vi "Panel.vi"(11 "StokePlotShortcuts in":refnum<class "RocketPlotShortcuts.lvclass">) -> ()   [LabVIEW 2021, in "RocketPlot.lvlib" / "RocketPlotShortcuts.lvclass"]
uses:
  RocketPlotShortcuts.lvclass
  C:/Program Files/National Instruments/LabVIEW 2021/user.lib/bjustice/TipStripOOPanel/Classes/TipPanel/TipPanel.lvclass
  C:/Program Files/National Instruments/LabVIEW 2021/vi.lib/IlluminatedG/IG OOPanel/OOPanel/Panel/Panel.lvclass
  <userlib>/bjustice/TipStripOOPanel/Classes/TipPanel/TipPanel.lvclass/TipPanel.ctl
  <userlib>/bjustice/TipStripOOPanel/Classes/TipPanel/Read New Panel UE.vi
  <vilib>/Futures/Futures/Promise/Promise.lvclass
  RocketPlotShortcuts.lvclass/RocketPlotShortcuts.ctl
  <vilib>/IlluminatedG/IG OOPanel/OOPanel/Panel/Panel.lvclass
  <userlib>/bjustice/TipStripOOPanel/Classes/TipPanel/TipPanel.lvclass
  <vilib>/IlluminatedG/IG OOPanel/OOPanel/OOPanel.lvlib
panel:
  # "Autosize\nall axes"
  # "Zoom in\ntime axis"
  # "Page\nUp"
  # "Zoom in\ny axis"
  # "Home"
  # "Insert"
  # "Right Click"
  # "Delta values"
  # "Middle Click"
  # "Right Click +Ctrl"
  # "Slive average"
  # "Pan"
  # "Left Click"
  # "Right Click +Shift"
  # "Plot names"
  # "Zoom out\ntime axis"
  # "Page\nDown"
  # "Zoom out\ny axis"
  # "Delete"
  # "Zoom to\nselection"
  # "Tool Tips"
  # "Wheel scroll"
  # "Zoom in/out"
  # "Pan\nin increments"
  # "Zoom actions apply\nto all axes"
  # "Shift"
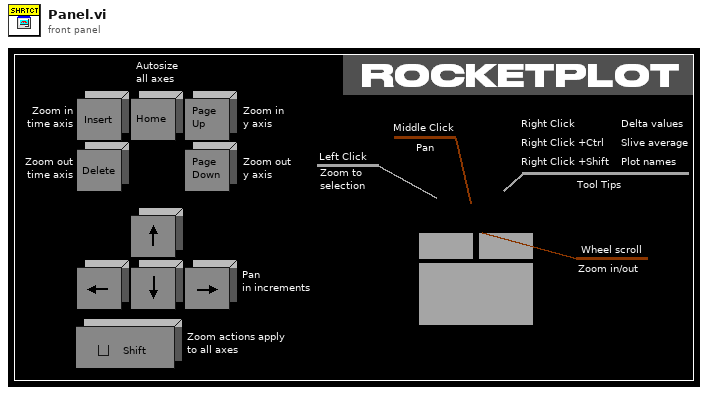
[diagram p1: front panel]
types:
  T1 = typedef "LVBoundsTypeDef.ctl" = cluster{"Width":u32, "Height":u32}
  T2 = typedef "OOPanel.lvlib/Panel.lvclass/Panel Events.ctl" = cluster{"Visbility":refnum<user-event>, "Close":refnum<user-event>}
  T3 = typedef "OOPanel.lvlib/Visibility State.ctl" = enum16{"Idle", "Closed", "Hidden", "Visible", "Subpanel", "Hidden Subpanel"}
  T4 = typedef "TipStrip2.lvlib/TipPanel.lvclass/ToPanelUE.ctl" = cluster{"TipPanel":refnum<class>, "Promise.Size":refnum<class "Promise.lvclass">}
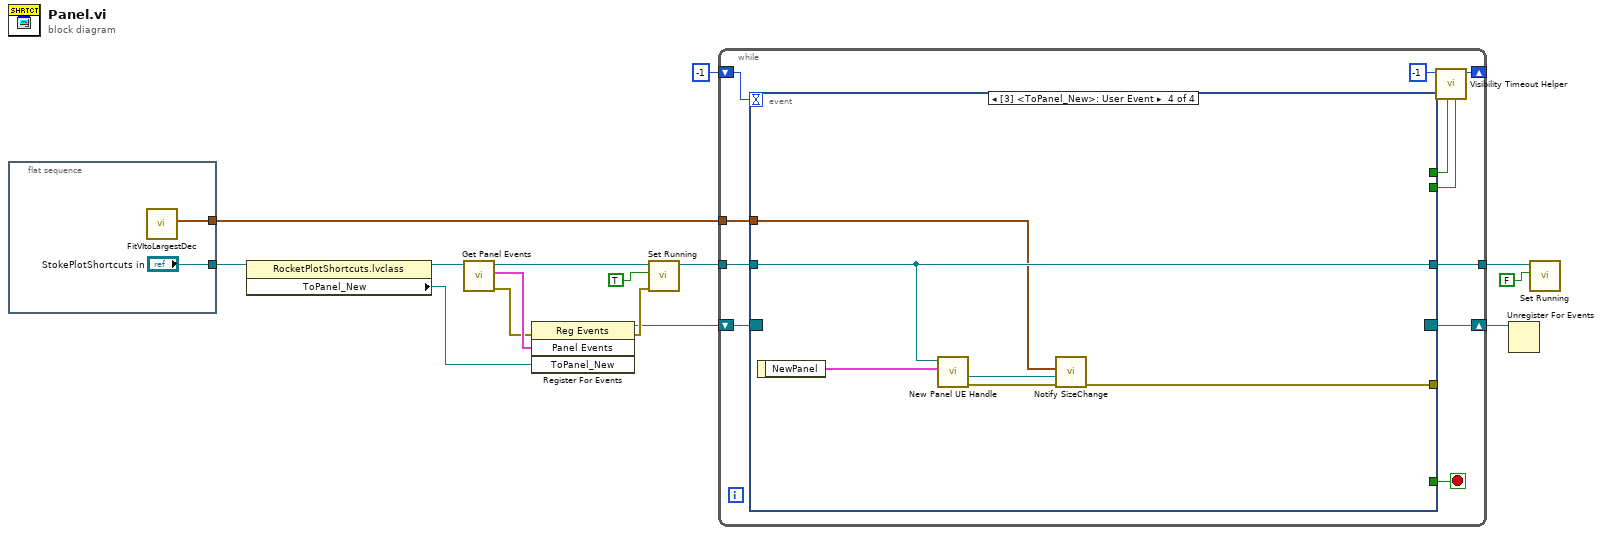
[diagram p0: block diagram]
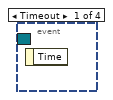
[diagram p2: hidden frame]
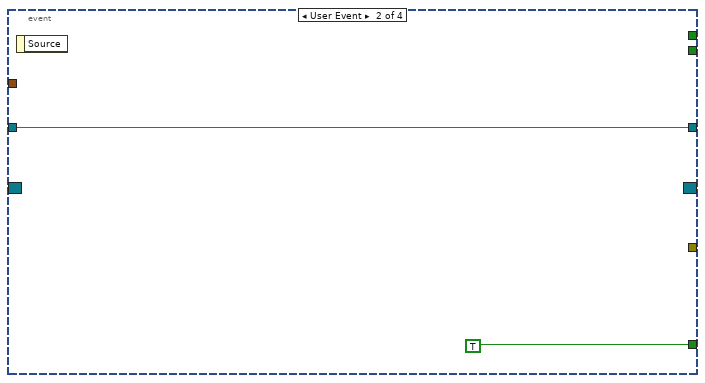
[diagram p3: hidden frame]
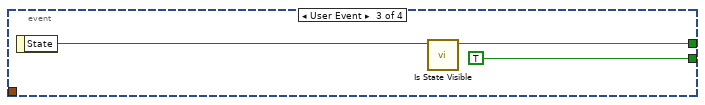
[diagram p4: hidden frame]
diagram:
  n1 = flat-sequence {
    tunnel: ["StokePlotShortcuts in"] -> w4
    tunnel: [w16] -> w1
    frame #0 {
      n2 = call "FitVItoLargestDec.vi"() -> ("content size"=w16:T1)  [unwired: 9 in, 2 out]
    }
  }
  n3 = property class="RocketPlotShortcuts.lvclass"(reference=w4) -> (reference out=w2:refnum<class "RocketPlotShortcuts.lvclass">, "ToPanel_New"=w3:refnum<user-event>)  [unwired: 1 in, 1 out]
  n4 = call <vilib>:"Get Panel Events.vi"("Panel in"=w2) -> ("error out"=w5:errorcluster, "Panel Events"=w15:T2, "Panel out"=w14:refnum<class "RocketPlotShortcuts.lvclass">)  [unwired: 8 in]
  n5 = register-events(error in=w5, w15, w3) -> (reference out=w11:refnum<event-registration>, error out=w12:errorcluster)  [unwired: 1 in]
  n6 = call <vilib>:"Set Running.vi"("error in (no error)"=w12, "Running"=TRUE, "Panel in"=w14) -> ("Panel out"=w10:refnum<class "RocketPlotShortcuts.lvclass">)  [unwired: 7 in, 1 out]
  n7 = while {
    shift-right: [w24] -> w7
    shift-left: w11 -> [w25]
    shift-right: [w27] -> _
    shift-left: -1 ("Timeout") -> [w26]
    tunnel: w10 -> [w20]
    tunnel: [w19] -> w6
    tunnel: w1 -> [w18]
    stop <- w21 stop-if-true
    n8 = event shown="[3] <ToPanel_New>: User Event" {
      selector: w25 -> [_ _ _ _]
      dyn-events: [_ _ _ _] -> w24
      timeout: w26 -> [_ _ _ _]
      tunnel: [_ _ w32 _] -> w23
      tunnel: [_ _ TRUE _] -> w22
      tunnel: [_ TRUE _ _] -> w21
      tunnel: w20 -> [_ w29 _ w37]
      tunnel: [_ w29 _ w37] -> w19
      tunnel: [_ _ _ w38] -> _
      tunnel: w18 -> [_ _ _ w34]
      event Timeout {
        n9 = event-data() -> ()  [unwired: 1 in, 1 out]
      }
      event User Event {
        n10 = event-data() -> ()  [unwired: 1 in, 1 out]
      }
      event User Event {
        n11 = event-data() -> ("State"=w33:T3)  [unwired: 1 in]
        n12 = call <vilib>:"Is State Visible.vi"("Visibility"=w33) -> ("Visible"=w32:bool)  [unwired: 10 in]
      }
      event User Event {
        n13 = event-data() -> ("NewPanel"=w39:T4)  [unwired: 1 in]
        n14 = call <userlib>:"New Panel UE Handle.vi"("NewPanel"=w39, "TipPanel in"=w37) -> ("error out"=w35:errorcluster, "Promise.Size"=w36:refnum<class "Promise.lvclass">)  [unwired: 7 in, 1 out]
        n15 = call <userlib>:"Notify SizeChange.vi"("error in (no error)"=w35, "Promise in"=w36, "content size"=w34) -> ("error out"=w38:errorcluster)  [unwired: 8 in]
      }
    }
    n16 = call <vilib>:"Visibility Timeout Helper.vi"("Update?"=w22, "Use Timeout?"=w23, "Visible Timeout mS"=-1) -> ("Timeout"=w27:i32)  [unwired: 8 in]
  }
  n17 = Unregister For Events(event registration refnum=w7) -> ()  [unwired: 1 in, 1 out]
  n18 = call <vilib>:"Set Running.vi"("Running"=FALSE, "Panel in"=w6) -> ()  [unwired: 8 in, 2 out]
